vi "Load SMU.vi"(7 "Load SMU Channel":string, 8 "error in (no error)":errorcluster, 9 "Current Limit":dbl, 10 "Voltage Level":dbl, 11 "IVI Refnum in":refnum<k15>) -> (0 "error out":errorcluster, 2 "Numeric":dbl, 3 "Numeric 2":dbl)   [LabVIEW 2021, in "Main T3.lvlib"]
uses:
  <instrlib>/niDCPower/nidcpower.llb/niDCPower Source Mode.ctl
  <instrlib>/niDCPower/nidcpower.llb/niDCPower Output Function.ctl
  Main T3.lvlib
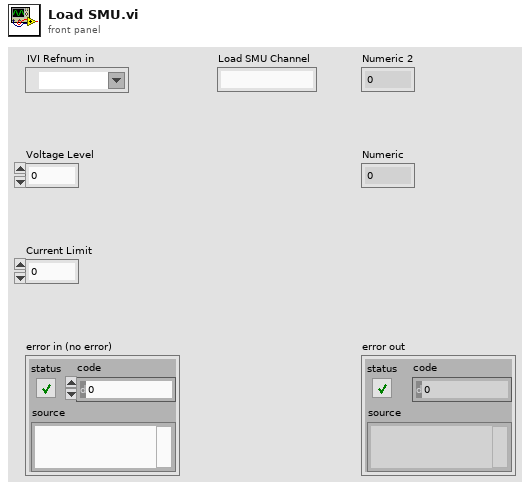
[diagram p1: front panel]
types:
  T1 = typedef "niDCPower Output Function.ctl" = i32
  T2 = typedef "niDCPower Source Mode.ctl" = i32
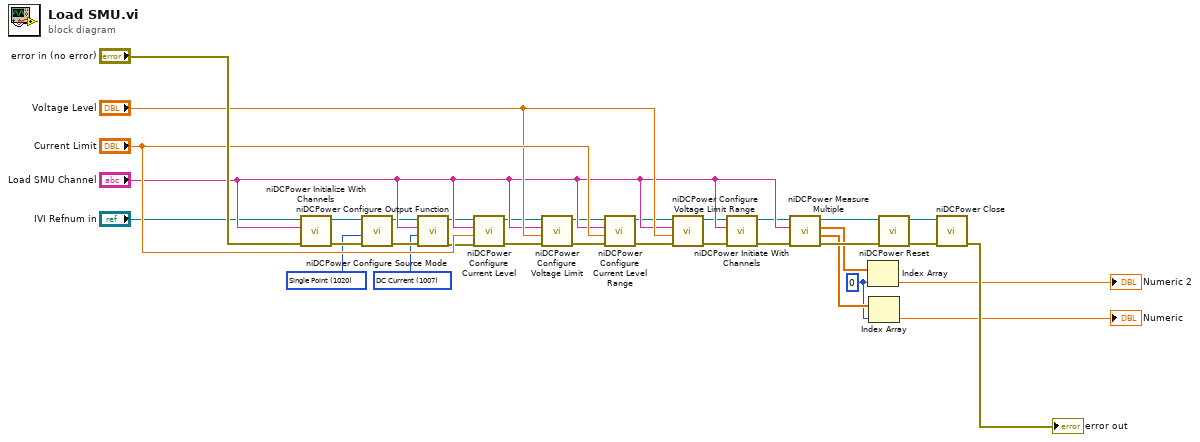
[diagram p0: block diagram]
diagram:
  w1 = T1 1007 items=["DC Voltage"=1006, "DC Current"=1007, "Pulse Voltage"=1049, "Pulse Current"=1050] ("output function")
  w10 = 0 ("index")
  w19 = T2 1020 items=["Single Point"=1020, "Sequence"=1021] ("source mode")
  n1 = call <instrlib>:"niDCPower Initialize With Channels.vi"("error in (no error)"="error in (no error)", "channels"="Load SMU Channel", "resource name"="IVI Refnum in") -> ("error out"=w23:errorcluster, "instrument handle out"=w22:refnum<k15>)  [unwired: 2 in, 5 out]
  n2 = call <instrlib>:"niDCPower Configure Source Mode.vi"("error in (no error)"=w23, "source mode"=w19, "instrument handle"=w22) -> ("error out"=w21:errorcluster, "instrument handle out"=w20:refnum<k15>)  [unwired: 7 out]
  n3 = call <instrlib>:"niDCPower Configure Output Function.vi"("error in (no error)"=w21, "output function"=w1, "channel name"="Load SMU Channel", "instrument handle"=w20) -> ("error out"=w3:errorcluster, "instrument handle out"=w2:refnum<k15>)  [unwired: 6 out]
  n4 = call <instrlib>:"niDCPower Configure Current Level.vi"("error in (no error)"=w3, "current level"="Current Limit", "channel name"="Load SMU Channel", "instrument handle"=w2) -> ("error out"=w26:errorcluster, "instrument handle out"=w27:refnum<k15>)  [unwired: 6 out]
  n5 = call <instrlib>:"niDCPower Configure Voltage Limit.vi"("error in (no error)"=w26, "voltage limit"="Voltage Level", "channel name"="Load SMU Channel", "instrument handle"=w27) -> ("error out"=w18:errorcluster, "instrument handle out"=w17:refnum<k15>)  [unwired: 6 out]
  n6 = call <instrlib>:"niDCPower Configure Current Level Range.vi"("error in (no error)"=w18, "current level range"="Current Limit", "channel name"="Load SMU Channel", "instrument handle"=w17) -> ("error out"=w16:errorcluster, "instrument handle out"=w15:refnum<k15>)  [unwired: 6 out]
  n7 = call <instrlib>:"niDCPower Configure Voltage Limit Range.vi"("error in (no error)"=w16, "voltage limit range"="Voltage Level", "channel name"="Load SMU Channel", "instrument handle"=w15) -> ("error out"=w6:errorcluster, "instrument handle out"=w7:refnum<k15>)  [unwired: 6 out]
  n8 = call <instrlib>:"niDCPower Initiate With Channels.vi"("error in (no error)"=w6, "channel name"="Load SMU Channel", "instrument handle"=w7) -> ("error out"=w4:errorcluster, "instrument handle out"=w5:refnum<k15>)  [unwired: 7 in]
  n9 = call <instrlib>:"niDCPower Measure Multiple.vi"("error in (no error)"=w4, "channel name"="Load SMU Channel", "instrument handle"=w5) -> ("error out"=w13:errorcluster, "current measurements"=w11:dbl[], "voltage measurements"=w12:dbl[], "instrument handle out"=w14:refnum<k15>)  [unwired: 5 out]
  n10 = Index Array(array=w12, index=w10) -> (element=→"Numeric 2":dbl)
  n11 = Index Array(array=w11, index=w10) -> (element=→"Numeric":dbl)
  n12 = call <instrlib>:"niDCPower Reset.vi"("error in (no error)"=w13, "instrument handle"=w14) -> ("error out"=w24:errorcluster, "instrument handle out"=w25:refnum<k15>)  [unwired: 2 in, 6 out]
  n13 = call <instrlib>:"niDCPower Close.vi"("error in (no error)"=w24, "instrument handle"=w25) -> ("error out"=→"error out":errorcluster)  [unwired: 9 out]
